vi "DtCreateCtrOneShotRepeatChan.vi"(1 "Requested\nPulse Width  (msecs)":dbl=1.0, 2 "Pulse Polarity":i32(ring)=600 items=["HighToLow"=600, "LowToHigh"=601], 5 "Board Name":string, 7 "Counter Num":u32, 9 "Trigger":i32(ring) items=["RisingEdge", "FallingEdge"], 11 "error in (no error)":errorcluster) -> (4 "Task out":i32, 6 "Actual Pulse \nWidth  (msecs)":dbl, 15 "error out":errorcluster)   [LabVIEW 2016]
doc: "Creates one or more virtual counter/timer channels that output a single pulse for a specified duration (in milliseconds) each time that the device detects a trigger (determined by the counter/timer's gate input signal). This type of task is also known as repetitive one-shot.\n\nYou can use a repetitive one-shot task to clean up a poor clock input signal by changing its pulse width, then outputting it.\n\nOnce you have created a virtual counter/timer channel for a repetitive one-shot task, use the DtOLStart VI to start the task."
uses:
  <userlib>/LV-Link3/DtLvLink.lvlib
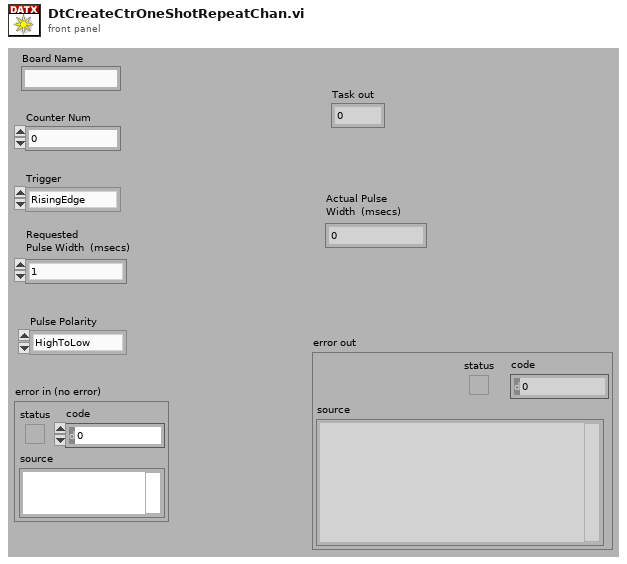
[diagram p1: front panel]
types:
  T1 = enum32{"AnalogInput", "AnalogOutput", "DigitalInput", "DigitalOutput", "Quadrature", "CounterTimer"}
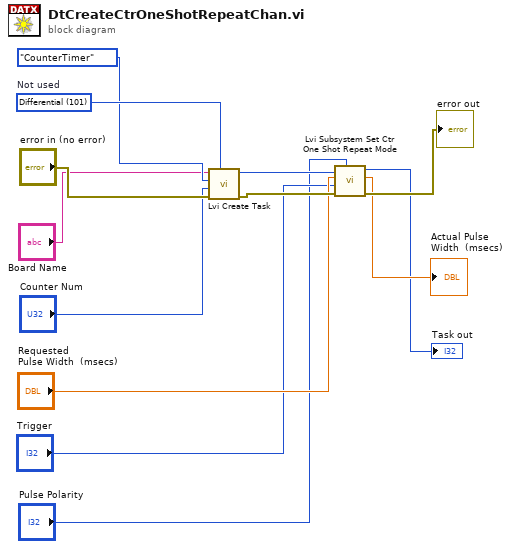
[diagram p0: block diagram]
diagram:
  w13 = 101 items=["SingleEnded"=100, "Differential"=101]  # Not used
  n1 = call <userlib>:"Lvi Create Task.vi"("SEorDiff"=w13, "error in (no error)"="error in (no error)", "SubSysIndex"="Counter Num", "ChanType"=T1."CounterTimer", "BoardName"="Board Name") -> ("error out"=w7:errorcluster, "TaskRef"=w4:i32)  [unwired: 4 in, 1 out]
  n2 = call <userlib>:"Lvi Subsystem Set Ctr One Shot Repeat Mode.vi"("Polarity"="Pulse Polarity", "error in (no error)"=w7, "GateEdge"="Trigger", "Millisecs"="Requested\nPulse Width  (msecs)", "TaskRef"=w4) -> ("error out"=→"error out":errorcluster, "ActualMillisecs"=→"Actual Pulse \nWidth  (msecs)":dbl, "TaskRef out"=→"Task out":i32)  [unwired: 3 in, 1 out]
